vi "SVX Orbit and Timebase Plot.vi"   [LabVIEW 2017, in "SoundVib_MCMDisplay.lvlib"]
doc: "Prepares unfiltered or filtered orbit plot data or timebase plot data for displaying on an Orbit Plot or Timebase Plot. Use this VI to prepare magnitude and phase data for entry into an orbit or timebase plot. Wire data to the <B>even-angle signals</B> input to determine the polymorphic instance to use or manually select the instance."
uses:
  <vilib>/addons/Sound and Vibration/Order Analysis/Data Presentation/SoundVib_MCMDisplay.lvlib
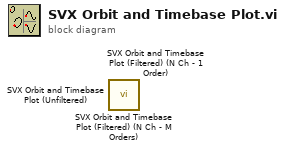
[diagram p0: block diagram]
diagram:
  n1 = call <vilib>:"SVX Orbit and Timebase Plot (Filtered) (N Ch - M Orders).vi"() -> ()  [unwired: 12 in, 4 out]
  n2 = call <vilib>:"SVX Orbit and Timebase Plot (Filtered) (N Ch - 1 Order).vi"() -> ()  [unwired: 12 in, 4 out]
  n3 = call <vilib>:"SVX Orbit and Timebase Plot (Unfiltered).vi"() -> ()  [unwired: 12 in, 4 out]
